vi "Form_设备通讯配置.vi"(11 "Module Admin":refnum<class "lib_QMH_Module_Admin.lvclass">) -> ()   [LabVIEW 2018]
uses:
  Basic Library/Module Admin_class/lib_QMH_Module_Admin.lvclass
  <vilib>/Utility/miscctls.llb/LVPointTypeDef.ctl
  <vilib>/Delacor/Delacor QMH/Libraries/Message Queue_class/Delacor_lib_QMH_Message Queue.lvclass/Delacor_lib_QMH_Message Queue.ctl
  Basic Library/Module Admin_class/lib_QMH_Module_Admin.lvclass/lib_QMH_Module_Admin.ctl
  <vilib>/Delacor/Delacor QMH/Libraries/Message Queue_class/Delacor_lib_QMH_Enqueue Message (Single).vi
  <vilib>/Utility/error.llb/Error Cluster From Error Code.vi
  <vilib>/ErrorRing/Error Ring.xnode
  <vilib>/Delacor/Delacor QMH/Libraries/Message Queue_class/Delacor_lib_QMH_Message Queue.lvclass
  Libraries/DAQ/DAQ.lvlib
panel:
  in  "IP协议":enum32{"IPV4", "IPV6"}(radio)
  in  "Connection Timeout":dbl
  in  "OK":bool caption="确认"
  in  "通信表索引":u16(ring) caption="通信设备" items=["LB-A1", "LB-A2"]
  in  "本机 IP（参考）":string
  in  "设置本机IP":bool
  in  "本机IP下拉列表":u16(ring) caption="本机 IP" items=["192.168.80.1", "192.168.44.1", "192.168.5.160"]
  in  "在网检测":bool caption="通讯检测"
  in  "断线重连":bool=TRUE caption="断线自动重连"
  in  "Protocol":enum16{"Serial Port", "Modbus TCP/IP"}(ring) caption="通讯方式"
  in  "选项卡控件":enum32{"Serial Port", "TCP/IP"}(tab) caption="Serial Settings"
  in  "RS485":T1={"Serial Port"="", "Unit ID"=1, "Baud Rate"=enum."19200", "Mode"=enum."RTU", "Parity"=0} {"Parity" items=["None", "Odd", "Even"]}
  in  "TCP":cluster{"IP Address":string, "Port (502)":u16}={"IP Address"="", "Port (502)"=502}
  in  "Apply":bool caption="应用"
  in  "Cancel":bool caption="取消"
  # "[ms]"
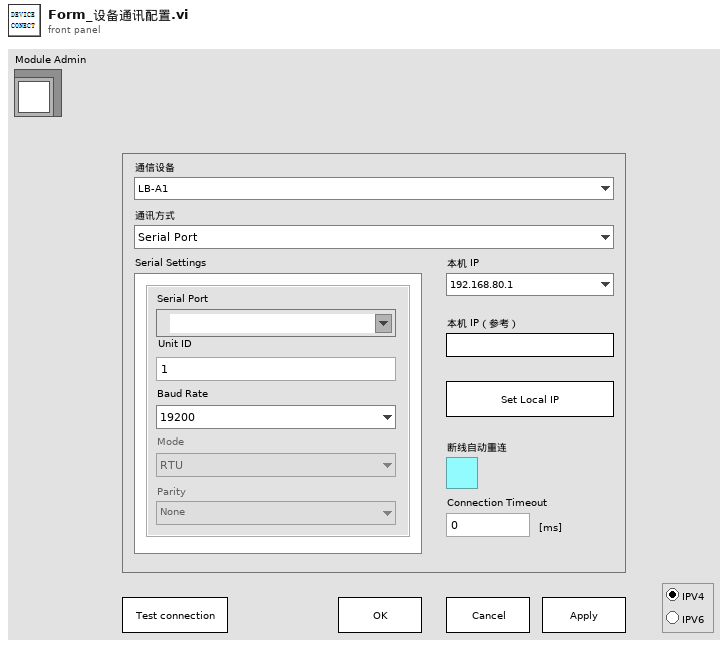
[diagram p1: front panel]
types:
  T1 = cluster{"Serial Port":refnum<visa-resource-name>, "Unit ID":u8, "Baud Rate":enum32{"1200", "2400", "4800", "9600", "19200", "38400", "57600", "115200"}, "Mode":enum16{"RTU", "ASCII"}, "Parity":u16}
  T2 = cluster{"name":string, "appended path":path, "通信表索引":refnum<vi>, "本机IP下拉列表":refnum<vi>, "Protocol":refnum<vi>, "选项卡控件":refnum<vi>, "RS485":refnum<vi>, "TCP":refnum<vi>, "本机 IP（参考）":refnum<vi>, "设置本机IP":refnum<vi>, "断线重连":refnum<vi>}
  T3 = typedef "LVPointTypeDef.ctl" = cluster{"Horizontal":i16, "Vertical":i16}
  T4 = cluster{"COM端口":refnum<visa-resource-name>, "站号":u8, "Baud Rate":enum32{"1200", "2400", "4800", "9600", "19200", "38400", "57600", "115200"}, "串口类型":enum16{"RTU", "ASCII"}, "校验":u16}
  T5 = cluster{"Serial Port":refnum<visa-resource-name>, "Baud Rate":enum32{"1200", "2400", "4800", "9600", "19200", "38400", "57600", "115200"}, "Mode":enum16{"RTU", "ASCII"}, "Parity":u16, "Unit ID":u8, "address":string, "port (502)":u16}
  T6 = enum8{"Enabled", "Disabled", "Disabled and Grayed Out"}
  T7 = cluster{"Unit ID":u8, "IP Address":string, "Port":u16, "Serial Port":string, "baud rate (9600)":u32, "Protocol":enum16{"Serial Port", "Modbus TCP/IP"}}
  T8 = cluster{"设备站号":u8, "IP Addr":string, "Port":u16, "COM":string, "baud rate (9600)":u32, "Protocol":enum16{"Serial Port", "Modbus TCP/IP"}}
  T9 = enum32{"1200", "2400", "4800", "9600", "19200", "38400", "57600", "115200"}
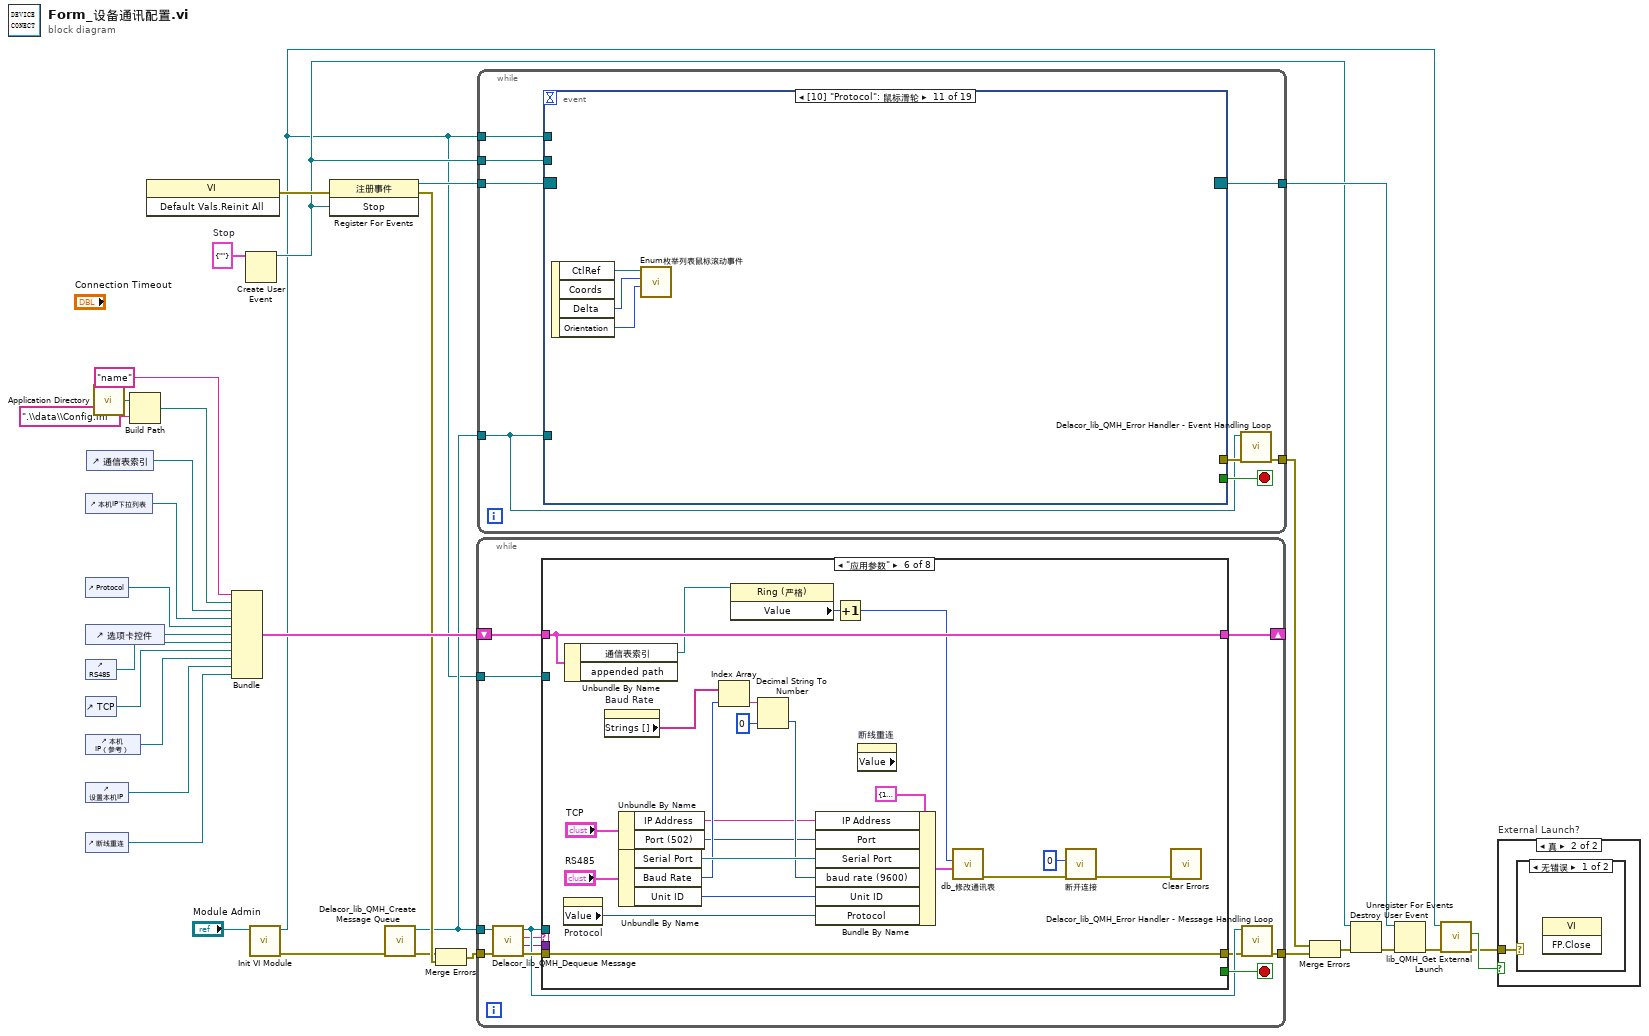
[diagram p0: block diagram]
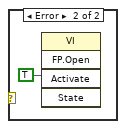
[diagram p3: hidden frame]
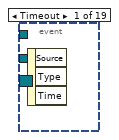
[diagram p4: hidden frame]
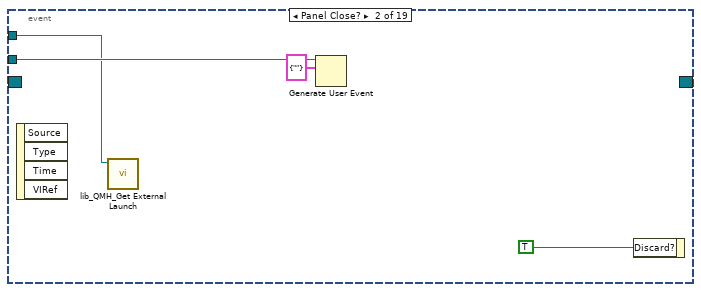
[diagram p5: hidden frame]
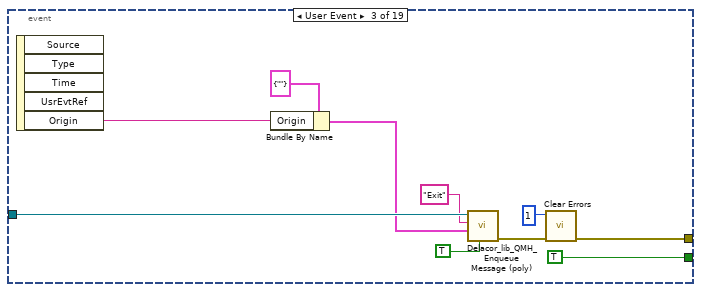
[diagram p6: hidden frame]
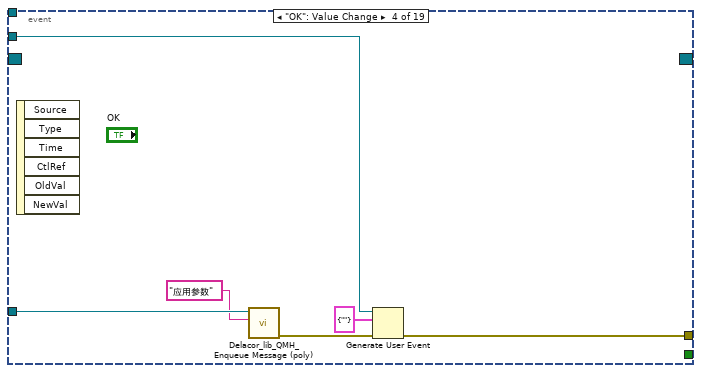
[diagram p7: hidden frame]
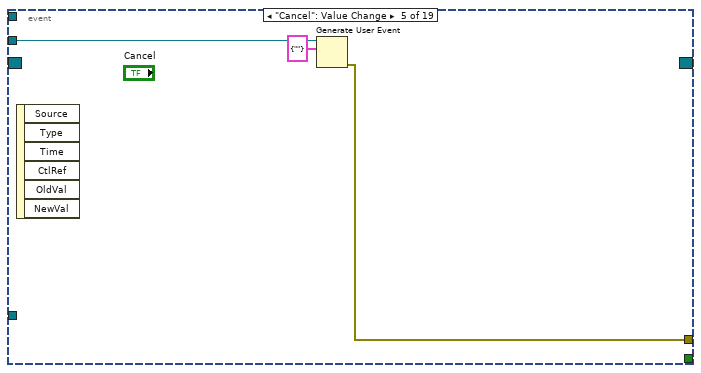
[diagram p8: hidden frame]
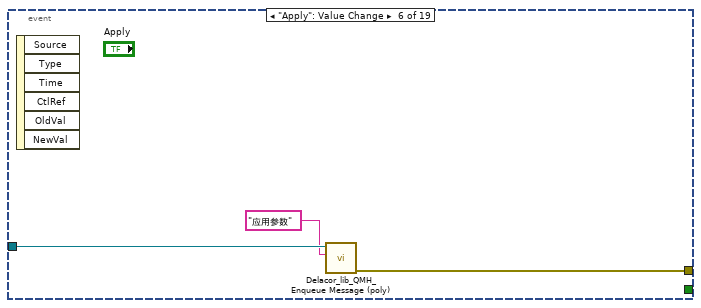
[diagram p9: hidden frame]
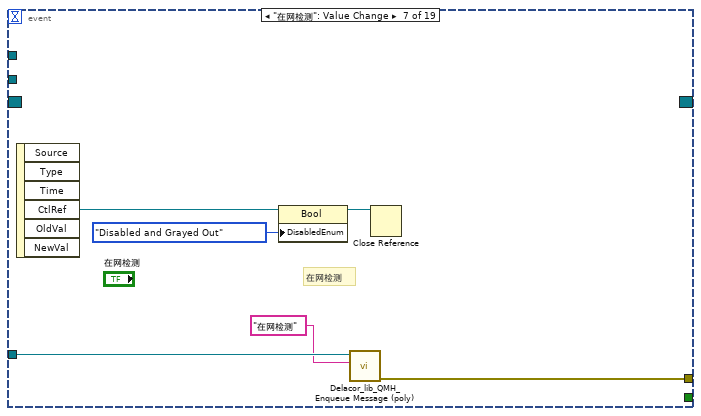
[diagram p10: hidden frame]
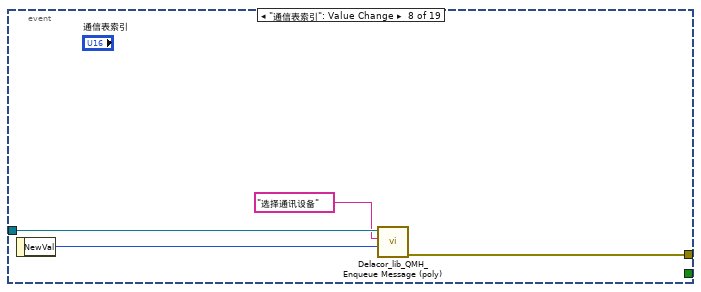
[diagram p11: hidden frame]
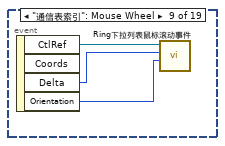
[diagram p12: hidden frame]
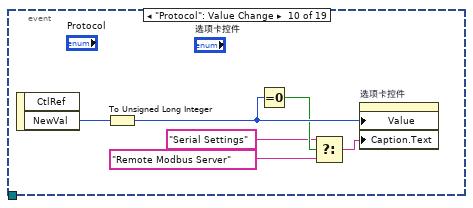
[diagram p13: hidden frame]
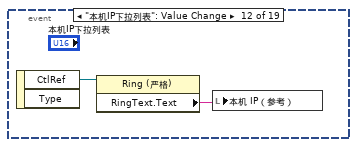
[diagram p14: hidden frame]
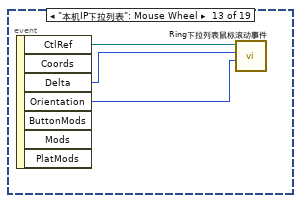
[diagram p15: hidden frame]
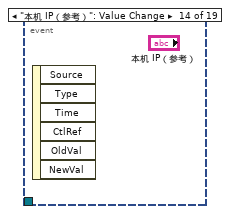
[diagram p16: hidden frame]
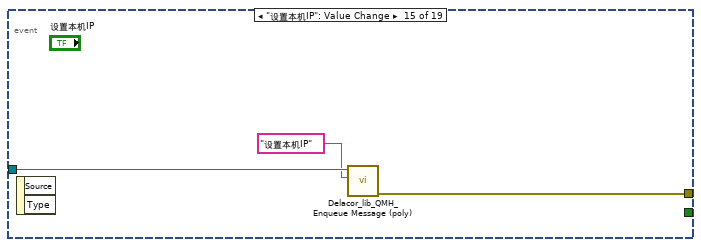
[diagram p17: hidden frame]
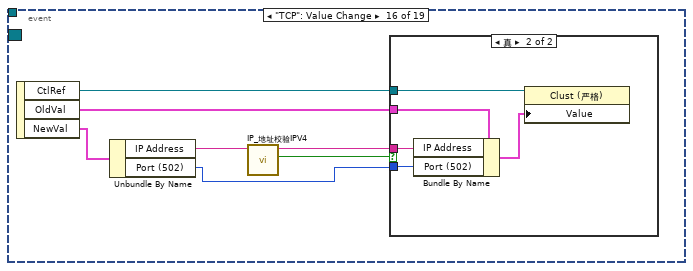
[diagram p18: hidden frame]
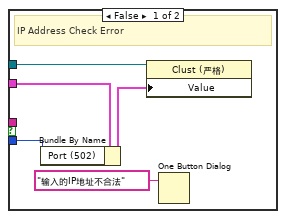
[diagram p19: hidden frame]
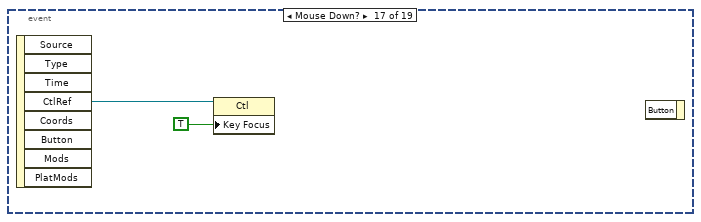
[diagram p20: hidden frame]
diagram:
  w22 = cluster{"Origin":string} {"Origin"=""}  # Stop
  n1 = control-ref of="本机IP下拉列表"() -> (w16:refnum<vi>)
  n2 = control-ref of="Protocol"() -> (w29:refnum<vi>)
  n3 = control-ref of="选项卡控件"() -> (w28:refnum<vi>)
  n4 = control-ref of="RS485"() -> (w27:refnum<vi>)
  n5 = control-ref of="TCP"() -> (w26:refnum<vi>)
  n6 = control-ref of="本机 IP（参考）"() -> (w25:refnum<vi>)
  n7 = control-ref of="设置本机IP"() -> (w24:refnum<vi>)
  n8 = control-ref of="断线重连"() -> (w23:refnum<vi>)
  n9 = control-ref of="通信表索引"() -> (w15:refnum<vi>)
  n10 = call <vilib>:"Application Directory.vi"() -> ("Application Directory"=w13:path)
  n11 = Build Path(base path=w13, name or relative path=".\\data\\Config.ini" ("名称或相对路径")) -> (appended path=w12:path)
  n12 = invoke class="VI" method="Default Vals.Reinit All"() -> (error out=w17:errorcluster)  [unwired: 3 in, 2 out]
  n13 = Bundle("name"="name", "appended path"=w12, "通信表索引"=w15, "本机IP下拉列表"=w16, "Protocol"=w29, "选项卡控件"=w28, "RS485"=w27, "TCP"=w26, "本机 IP（参考）"=w25, "设置本机IP"=w24, "断线重连"=w23) -> (w30:T2)  [unwired: 1 in]
  n14 = Create User Event(user event datatype=w22) -> (user event=w3:refnum<user-event>)  [unwired: 1 in, 1 out]
  n15 = call "Init VI Module.vi"("Module Admin in"="Module Admin") -> ("error out"=w11:errorcluster, "Module Admin out"=w2:refnum<class "lib_QMH_Module_Admin.lvclass">)  [unwired: 9 in]
  n16 = register-events(error in=w17, w3) -> (reference out=w31:refnum<event-registration>, error out=w20:errorcluster)  [unwired: 1 in]
  n17 = call <vilib>:"Delacor_lib_QMH_Create Message Queue.vi"("error in"=w11) -> ("error out"=w18:errorcluster, "Message Queue"=w19:refnum<class "Delacor_lib_QMH_Message Queue.lvclass">)  [unwired: 9 in]
  n18 = Merge Errors(w18, w20) -> (w21:errorcluster)
  n19 = while {
    tunnel: w19 -> [w41]
    tunnel: w21 -> [w42]
    tunnel: [w35] -> w33
    shift-right: [w44] -> _
    shift-left: w30 -> [w43]
    tunnel: w2 -> [w34]
    stop <- w45 stop-if-true
    n20 = call-dynamic "Delacor_lib_QMH_Dequeue Message.vi"("error in"=w42, "Message Queue in"=w41) -> ("error out"=w40:errorcluster, "Message Data"=w37:variant, "Message"=w38:string, "Message Queue out"=w39:refnum<class "Delacor_lib_QMH_Message Queue.lvclass">)  [unwired: 6 in]
    n21 = case shown="\"应用参数\"" w38 {
      selector: w38 -> [w50 _ _ _ _ _ _ _]
      tunnel: w39 -> [_ w64 _ _ _ _ w162 w172]
      tunnel: w40 -> [w47 w63 w101 w106 w136 w156 w167 w177]
      tunnel: w37 -> [_ _ w99 _ _ _ w168 w178]
      tunnel: [_ _ _ _ _ _ _ TRUE] -> w45
      tunnel: [w46 w62 w100 w106 w136 w156 w163 w171] -> w36
      tunnel: [w49 w73 w97 w102 w135 w158 w169 w173] -> w44
      tunnel: w43 -> [w49 w73 w97 w102 w135 w158 w169 w173]
      tunnel: w34 -> [_ _ _ _ _ _ _ _]
      frame "", Default {
        n22 = Unbundle By Name(w49) -> ("name"=w48:string)
        n23 = xnode "错误下拉列表"("参数 0"=w50, "参数 1"=w48) -> ("错误输出"=w51:errorcluster)
        n24 = Merge Errors(w47, w51) -> (w46:errorcluster)
      }
      frame "Initialize" {
        w60 = u16 0 ("值")
        n25 = Unbundle By Name(w73) -> ("本机IP下拉列表"=w72:refnum<vi>, "本机 IP（参考）"=w68:refnum<vi>, "通信表索引"=w66:refnum<vi>)
        n26 = String To IP(1:"" ("名称")) -> (0:w70:u32[])
        n27 = call "db_查询通讯设备名称列表.vi"() -> ("通讯设备列表名"=w65:string[])  [unwired: 10 in, 1 out]
        n28 = for {
          tunnel: w70 -> [w77] mode=indexing
          tunnel: [w75] -> w69 mode=indexing
          n29 = IP To String(1:TRUE ("句点符号？(F)"), 2:w77) -> (0:w75:string)
        }
        n30 = property class="Ring (严格)"(reference=w66, "Strings []"=w65, "Value"=w60) -> ()  [unwired: 1 in, 2 out]
        n31 = call-poly <vilib>:"Delacor_lib_QMH_Enqueue Message (poly).vi"("error in"=w63, "Message Data"=w60, "Message"="选择通讯设备", "Message Queue in"=w64) -> ("error out"=w62:errorcluster)  [unwired: 6 in, 1 out]
        n32 = property class="Ring (严格)"(reference=w72, "Strings []"=w69) -> ("RingText.Text"=w67:string)  [unwired: 1 in, 2 out]
        n33 = property class="Str"(reference=w68, "Text.Text"=w67) -> ()  [unwired: 1 in, 2 out]
        n34 = property on="窗格" class="Pane"("Origin"=T3 {"Horizontal"=0, "Vertical"=0} ("原点")) -> ()  [unwired: 2 in, 2 out]
      }
      frame "选择通讯设备" {
        n35 = Unbundle By Name(w97) -> ("TCP"=w96:refnum<vi>, "RS485"=w95:refnum<vi>, "Protocol"=w94:refnum<vi>)  [unwired: 1 out]
        n36 = Variant To Data(error in=w101, type=0, Variant=w99) -> (data=w88:i32, error out=w100:errorcluster)
        n37 = Increment(x=w88) -> (x+1=w82:i32)
        n38 = property on="Baud Rate" class="Enum (严格)"() -> ("Strings []"=w92:string[])  [unwired: 2 in, 2 out]
        n39 = call "db_查询通讯表.vi"("ID"=w82) -> ("设备通讯参数"=w87:T8)  [unwired: 9 in, 1 out]
        n40 = Unbundle By Name(w87) -> ("IP Addr"=w78:string, "Port"=w80:u16, "COM"=w93:string, "baud rate (9600)"=w91:u32, "设备站号"=w85:u8, "Protocol"=w86:enum16{"Serial Port", "Modbus TCP/IP"})
        n41 = Number To Decimal String(number=w91) -> (decimal integer string=w90:string)  [unwired: 1 in]
        n42 = Search 1D Array(1D array=w92, element=w90) -> (index of element=w89:i32)  [unwired: 1 in]
        n43 = Bundle By Name(cluster=cluster{"IP Address":string, "Port (502)":u16} {"IP Address"="", "Port (502)"=0} ("值"), "IP Address"=w78, "Port (502)"=w80) -> (w81:cluster{"IP Address":string, "Port (502)":u16})
        n44 = Bundle By Name(cluster=T4 {"COM端口"="", "站号"=0, "Baud Rate"=enum."1200", "串口类型"=enum."RTU", "校验"=0} ("值"), "COM端口"=w93, "Baud Rate"=w89, "站号"=w85) -> (w83:T4)
        n45 = property on="属性节点" class="Enum (严格)"(reference=w94, "Val(Sgnl)"=w86) -> ()  [unwired: 1 in, 2 out]
        n46 = property class="Clust (严格)"(reference=w95, "Value"=w83) -> ()  [unwired: 1 in, 2 out]
        n47 = property class="Clust (严格)"(reference=w96, "Value"=w81) -> ()  [unwired: 1 in, 2 out]
      }
      frame "设置本机IP" {
        n48 = Unbundle By Name(w102) -> ("本机 IP（参考）"=w105:refnum<vi>)
        n49 = property class="Str"(reference=w105) -> ("Value"=w104:string)  [unwired: 1 in, 2 out]
        n50 = call "IP_设置本机IP地址.vi"("IP模式"=enum16{"使用特定ip", "自动获取ip"}."使用特定ip", "IP Address"=w104) -> ()  [unwired: 7 in, 3 out]
      }
      frame "在网检测" {
        w127 = 128  # call and forget
        n51 = Unbundle By Name(w135) -> ("Protocol"=w134:refnum<vi>, "RS485"=w133:refnum<vi>, "TCP"=w132:refnum<vi>)
        n52 = property on="属性节点" class="Clust (严格)"(reference=w133) -> ("Value"=w116:T1)  [unwired: 1 in, 2 out]
        n53 = property on="属性节点" class="Clust (严格)"(reference=w132) -> ("Value"=w130:cluster{"IP Address":string, "Port (502)":u16})  [unwired: 1 in, 2 out]
        n54 = property on="属性节点" class="Enum (严格)"(reference=w134) -> ("Value"=w120:enum16{"Serial Port", "Modbus TCP/IP"})  [unwired: 1 in, 2 out]
        n55 = Unbundle By Name(w130) -> ("IP Address"=w110:string, "Port (502)"=w117:u16)
        n56 = Unbundle By Name(w116) -> ("Serial Port"=w113:refnum<visa-resource-name>, "Unit ID"=w112:u8, "Baud Rate"=w114:T9, "Mode"=w111:enum16{"RTU", "ASCII"}, "Parity"=w115:u16)
        n57 = vi-ref "Modbus Connection Test.vi"() -> (w121:refnum<vi>)
        n58 = Bundle By Name(cluster=T5 {"Serial Port"="", "Baud Rate"=enum."1200", "Mode"=enum."RTU", "Parity"=0, "Unit ID"=0, "address"="", "port (502)"=0} ("Modbus Info"), "Serial Port"=w113, "Baud Rate"=w114, "Mode"=w111, "Parity"=w115, "Unit ID"=w112, "address"=w110, "port (502)"=w117) -> (w118:T5)
        n59 = property class="VI"(reference=w121) -> (reference out=w109:refnum<vi>, error out=w128:errorcluster, "Path"=w129:path)  [unwired: 1 in]
        n60 = Open VI Reference(type specifier VI Refnum (for type only)=refnum<vi> refnum, vi path=w129, options=w127, error in (no error)=w128) -> (vi reference=w124:refnum<vi>, error out=w125:errorcluster)  [unwired: 2 in]
        n61 = call-by-ref "Start Asynchronous Call"(reference=w124, error in=w125, "Protocol"=w120, "Modbus Info"=w118) -> (reference out=w123:refnum<vi>, error out=w122:errorcluster)  [unwired: 9 in, 1 out]
        n62 = Close Reference(reference=w123, error in (no error)=w122) -> (error out=w108:errorcluster)
        n63 = Close Reference(reference=w109, error in (no error)=w108) -> (error out=w107:errorcluster)
        n64 = property on="在网检测" class="Bool"(error in=w107, "DisabledEnum"=T6."Enabled" ("禁用")) -> ()  [unwired: 1 in, 2 out]
      }
      frame "应用参数" {
        n65 = property on="Protocol" class="Enum (严格)"() -> ("Value"=w152:enum16{"Serial Port", "Modbus TCP/IP"})  [unwired: 2 in, 2 out]
        n66 = Unbundle By Name(w158) -> ("通信表索引"=w155:refnum<vi>)  [unwired: 1 out]
        n67 = property on="Baud Rate" class="Enum (严格)"() -> ("Strings []"=w148:string[])  [unwired: 2 in, 2 out]
        n68 = Unbundle By Name("TCP") -> ("IP Address"=w140:string, "Port (502)"=w143:u16)
        n69 = Unbundle By Name("RS485") -> ("Serial Port"=w154:refnum<visa-resource-name>, "Baud Rate"=w147:T9, "Unit ID"=w151:u8)
        n70 = Index Array(array=w148, index=w147) -> (element=w146:string)
        n71 = property class="Ring (严格)"(reference=w155) -> ("Value"=w144:u16)  [unwired: 1 in, 2 out]
        n72 = Decimal String To Number(string=w146, default (0L)=u32 0 ("默认(0 I32)")) -> (number=w149:u32)  [unwired: 1 in, 1 out]
        n73 = Bundle By Name(cluster=T7 {"Unit ID"=1, "IP Address"="127.0.0.1", "Port"=255, "Serial Port"="COM3", "baud rate (9600)"=9600, "Protocol"=enum."Serial Port"} ("设备通讯参数"), "IP Address"=w140, "Port"=w143, "Serial Port"=w154, "baud rate (9600)"=w149, "Unit ID"=w151, "Protocol"=w152) -> (w141:T7)
        n74 = Increment(x=w144) -> (x+1=w145:u16)
        n75 = property on="断线重连" class="Bool (严格)" props=["Value"]() -> ()  [unwired: 2 in, 3 out]
        n76 = call "db_修改通讯表.vi"("设备通讯参数"=w141, "id"=w145) -> ("error out"=w138:errorcluster)  [unwired: 8 in, 1 out]
        n77 = call "断开连接.vi"("error in"=w138, "Mod ID"=0) -> ("error out"=w137:errorcluster)  [unwired: 9 in]
        n78 = call <vilib>:"Clear Errors.vi"("error in (no error)"=w137) -> ()  [unwired: 5 in, 2 out]
      }
      frame "Error" {
        n79 = Variant To Data(error in=w167, type=errorcluster {"status"=FALSE, "code"=0, "source"=""} ("error constant"), Variant=w168) -> (data=w165:errorcluster, error out=w164:errorcluster)
        n80 = call <vilib>:"Simple Error Handler.vi"("error in (no error)"=w165) -> ()  [unwired: 4 in, 5 out]
        n81 = call-poly <vilib>:"Delacor_lib_QMH_Enqueue Message (poly).vi"("Priority Message? (F)"=TRUE, "Message"="Exit", "Message Queue in"=w162) -> ("error out"=w161:errorcluster)  [unwired: 7 in, 1 out]
        n82 = Merge Errors(w164, w161) -> (w163:errorcluster)
      }
      frame "Exit" {
        w179 = 91  # 91: not all Exit messages will have an argument
        n83 = Variant To Data(error in=w177, type=cluster{"Origin":string} {"Origin"=""}, Variant=w178) -> (data=w174:cluster{"Origin":string}, error out=w176:errorcluster)
        n84 = Unbundle By Name(w174) -> ()  [unwired: 1 out]
        n85 = call <vilib>:"Clear Errors.vi"("error in (no error)"=w176, "specific error code to clear (0: all)"=w179) -> ("error out"=w170:errorcluster)  [unwired: 4 in, 1 out]
        n86 = call-dynamic "Delacor_lib_QMH_Release Message Queue.vi"("error in"=w170, "Message Queue"=w172) -> ("error out"=w171:errorcluster)  [unwired: 9 in]
      }
    }
    n87 = call-dynamic "Delacor_lib_QMH_Error Handler - Message Handling Loop.vi"("error in"=w36, "Message Queue in"=w39) -> ("dup error in"=w35:errorcluster)  [unwired: 8 in, 1 out]
  }
  n88 = while {
    tunnel: w19 -> [w183]
    tunnel: [w182] -> w32
    tunnel: [w187] -> w4
    tunnel: w31 -> [w186]
    tunnel: w3 -> [w185]
    tunnel: w2 -> [w181]
    stop <- w188 stop-if-true
    n89 = event shown="[10] \"Protocol\": 鼠标滑轮" {
      selector: w186 -> [_ _ _ _ _ _ _ _ _ _ _ _ _ _ _ _ _ _ _]
      dyn-events: [_ _ _ _ _ _ _ _ _ _ _ _ _ _ _ _ _ _ _] -> w187
      timeout: _ -> [_ _ _ _ _ _ _ _ _ _ _ _ _ _ _ _ _ _ _]
      tunnel: [_ _ TRUE ("放弃？") _ _ _ _ _ _ _ _ _ _ _ _ _ _ _ _] -> w188
      tunnel: w183 -> [_ _ w197 w204 _ w214 w220 w224 _ _ _ _ _ _ w244 _ _ _ _]
      tunnel: [_ _ w200 w205 w209 w213 w219 w223 _ _ _ _ _ _ w243 _ _ _ _] -> w184
      tunnel: w185 -> [_ w191 _ w207 w211 _ _ _ _ _ _ _ _ _ _ _ _ _ _]
      tunnel: w181 -> [_ w189 _ _ _ _ _ _ _ _ _ _ _ _ _ _ _ _ _]
      event Timeout {
        n90 = event-data() -> ()  [unwired: 1 in, 3 out]
      }
      event Panel Close? {
        n91 = event-data() -> ()  [unwired: 1 in, 4 out]
        n92 = call "lib_QMH_Get External Launch.vi"("Module Admin in"=w189) -> ()  [unwired: 8 in, 3 out]
        n93 = Generate User Event(user event=w191, event data cluster=cluster{"Origin":string} {"Origin"=""} ("事件数据")) -> ()  [unwired: 2 in, 2 out]
        n94 = event-data("Discard?"=TRUE ("放弃？")) -> ()  [unwired: 1 in, 1 out]
      }
      event User Event {
        n95 = event-data() -> ("Origin"=w198:string)  [unwired: 1 in, 4 out]
        n96 = Bundle By Name(cluster=cluster{"Origin":string} {"Origin"=""}, "Origin"=w198) -> (w195:cluster{"Origin":string})
        n97 = call-poly <vilib>:"Delacor_lib_QMH_Enqueue Message (poly).vi"("Priority Message? (F)"=TRUE, "Message Data"=w195, "Message"="Exit", "Message Queue in"=w197) -> ("error out"=w193:errorcluster)  [unwired: 6 in, 1 out]
        n98 = call <vilib>:"Clear Errors.vi"("error in (no error)"=w193, "specific error code to clear (0: all)"=1) -> ("error out"=w200:errorcluster)  [unwired: 4 in, 1 out]
      }
      event "OK": Value Change {
        n99 = event-data() -> ()  [unwired: 1 in, 6 out]
        n100 = call-poly <vilib>:"Delacor_lib_QMH_Enqueue Message (poly).vi"("Message"="应用参数", "Message Queue in"=w204) -> ("error out"=w206:errorcluster)  [unwired: 8 in, 1 out]
        n101 = Generate User Event(user event=w207, event data cluster=cluster{"Origin":string} {"Origin"=""} ("事件数据"), error in=w206) -> (error out=w205:errorcluster)  [unwired: 1 in, 1 out]
      }
      event "Cancel": Value Change {
        n102 = event-data() -> ()  [unwired: 1 in, 6 out]
        n103 = Generate User Event(user event=w211, event data cluster=cluster{"Origin":string} {"Origin"=""} ("事件数据")) -> (error out=w209:errorcluster)  [unwired: 2 in, 1 out]
      }
      event "Apply": Value Change {
        n104 = event-data() -> ()  [unwired: 1 in, 6 out]
        n105 = call-poly <vilib>:"Delacor_lib_QMH_Enqueue Message (poly).vi"("Message"="应用参数", "Message Queue in"=w214) -> ("error out"=w213:errorcluster)  [unwired: 8 in, 1 out]
      }
      event "在网检测": Value Change {
        # "在网检测"
        n106 = event-data() -> ("CtlRef"=w216:refnum<vi>)  [unwired: 1 in, 5 out]
        n107 = property on="属性节点" class="Bool"(reference=w216, "DisabledEnum"=T6."Disabled and Grayed Out" ("禁用")) -> (reference out=w215:refnum<vi>)  [unwired: 1 in, 1 out]
        n108 = call-poly <vilib>:"Delacor_lib_QMH_Enqueue Message (poly).vi"("Message"="在网检测", "Message Queue in"=w220) -> ("error out"=w219:errorcluster)  [unwired: 8 in, 1 out]
        n109 = Close Reference(reference=w215) -> ()  [unwired: 1 in, 1 out]
      }
      event "通信表索引": Value Change {
        n110 = event-data() -> ("NewVal"=w221:u16)  [unwired: 1 in]
        n111 = call-poly <vilib>:"Delacor_lib_QMH_Enqueue Message (poly).vi"("Message Data"=w221, "Message"="选择通讯设备", "Message Queue in"=w224) -> ("error out"=w223:errorcluster)  [unwired: 7 in, 1 out]
      }
      event "通信表索引": Mouse Wheel {
        n112 = event-data() -> ("CtlRef"=w227:refnum<vi>, "Delta"=w226:i32, "Orientation"=w225:enum16{"Horizontal", "Vertical"})  [unwired: 1 in, 1 out]
        n113 = call "Ring下拉列表鼠标滚动事件.vi"("方向"=w225, "Delta"=w226, "CtlRef"=w227) -> ()  [unwired: 7 in, 2 out]
      }
      event "Protocol": Value Change {
        n114 = event-data() -> ("NewVal"=w233:enum16{"Serial Port", "Modbus TCP/IP"})  [unwired: 1 in, 1 out]
        n115 = To Unsigned Long Integer(number=w233) -> (unsigned 32bit integer=w232:u32)
        n116 = Equal To 0?(x=w232) -> (x = 0?=w231:bool)
        n117 = Select(t="Serial Settings" ("标题.文本"), s=w231, f="Remote Modbus Server" ("标题.文本")) -> (s? t:f=w228:string)
        n118 = property on="选项卡控件" class="TabCtl (严格)"("Value"=w232, "Caption.Text"=w228) -> ()  [unwired: 2 in, 2 out]
      }
      event "Protocol": Mouse Wheel {
        n119 = event-data() -> ("CtlRef"=w236:refnum<vi>, "Delta"=w235:i32, "Orientation"=w234:enum16{"Horizontal", "Vertical"})  [unwired: 1 in, 1 out]
        n120 = call "Enum枚举列表鼠标滚动事件.vi"("方向"=w234, "Delta"=w235, "CtlRef"=w236) -> ()  [unwired: 7 in, 2 out]
      }
      event "本机IP下拉列表": Value Change {
        n121 = event-data() -> ("CtlRef"=w238:refnum<vi>)  [unwired: 1 in, 1 out]
        n122 = property class="Ring (严格)"(reference=w238) -> ("RingText.Text"=w237:string)  [unwired: 1 in, 2 out]
        n123 = local write "本机 IP（参考）"(w237) -> ()
      }
      event "本机IP下拉列表": Mouse Wheel {
        n124 = event-data() -> ("CtlRef"=w241:refnum<vi>, "Delta"=w240:i32, "Orientation"=w239:enum16{"Horizontal", "Vertical"})  [unwired: 1 in, 4 out]
        n125 = call "Ring下拉列表鼠标滚动事件.vi"("方向"=w239, "Delta"=w240, "CtlRef"=w241) -> ()  [unwired: 7 in, 2 out]
      }
      event "本机 IP（参考）": Value Change {
        n126 = event-data() -> ()  [unwired: 1 in, 6 out]
      }
      event "设置本机IP": Value Change {
        n127 = event-data() -> ()  [unwired: 1 in, 2 out]
        n128 = call-poly <vilib>:"Delacor_lib_QMH_Enqueue Message (poly).vi"("Message"="设置本机IP", "Message Queue in"=w244) -> ("error out"=w243:errorcluster)  [unwired: 8 in, 1 out]
      }
      event "TCP": Value Change {
        n129 = event-data() -> ("CtlRef"=w246:refnum<vi>, "OldVal"=w249:cluster{"IP Address":string, "Port (502)":u16}, "NewVal"=w251:cluster{"IP Address":string, "Port (502)":u16})  [unwired: 1 in]
        n130 = Unbundle By Name(w251) -> ("IP Address"=w250:string, "Port (502)"=w245:u16)
        n131 = call "IP_地址校验IPV4.vi"("IP Address"=w250) -> ("合法？"=w248:bool, "所有匹配"=w247:string)  [unwired: 9 in]
        n132 = case shown="真" w248 {
          tunnel: w246 -> [w256 w261]
          tunnel: w249 -> [w255 w260]
          tunnel: w247 -> [_ w258]
          tunnel: w245 -> [w252 w257]
          frame False {
            # "IP Address Check Error"
            n133 = Bundle By Name(cluster=w255, "Port (502)"=w252) -> (w253:cluster{"IP Address":string, "Port (502)":u16})
            n134 = property class="Clust (严格)"(reference=w256, "Value"=w253) -> ()  [unwired: 1 in, 2 out]
            n135 = One Button Dialog(message="输入的IP地址不合法" ("消息")) -> ()  [unwired: 1 in, 1 out]
          }
          frame True {
            n136 = Bundle By Name(cluster=w260, "IP Address"=w258, "Port (502)"=w257) -> (w259:cluster{"IP Address":string, "Port (502)":u16})
            n137 = property class="Clust (严格)"(reference=w261, "Value"=w259) -> ()  [unwired: 1 in, 2 out]
          }
        }
      }
      event "TCP.IP Address", "TCP.Port (502)": Mouse Down? {
        n138 = event-data() -> ("CtlRef"=w262:refnum<vi>)  [unwired: 1 in, 7 out]
        n139 = property class="Ctl"(reference=w262, "Key Focus"=TRUE ("键选中")) -> ()  [unwired: 1 in, 2 out]
        n140 = event-data() -> ()  [unwired: 2 in, 1 out]
      }
      event "TCP.IP Address", "TCP.Port (502)": Mouse Move {
        n141 = event-data() -> ()  [unwired: 1 in, 5 out]
      }
      event "断线重连": Value Change {
        n142 = event-data() -> ()  [unwired: 1 in, 2 out]
      }
    }
    n143 = call-dynamic "Delacor_lib_QMH_Error Handler - Event Handling Loop.vi"("error in"=w184, "Message Queue in"=w183) -> ("dup error in"=w182:errorcluster)  [unwired: 8 in, 1 out]
  }
  n144 = Merge Errors(w32, w33) -> (w5:errorcluster)
  n145 = Destroy User Event(user event=w3, error in=w5) -> (error out=w9:errorcluster)
  n146 = Unregister For Events(event registration refnum=w4, error in=w9) -> (error out=w8:errorcluster)
  n147 = call "lib_QMH_Get External Launch.vi"("error in (no error)"=w8, "Module Admin in"=w2) -> ("error out"=w6:errorcluster, "External Launch"=w7:bool)  [unwired: 7 in, 1 out]
  n148 = case "External Launch?" shown="真" w7 {
    tunnel: w6 -> [_ w264]
    frame False {
    }
    frame True {
      n149 = case "条件结构" shown="无错误" w264 {
        frame No Error {
          n150 = invoke class="VI" method="FP.Close"() -> ()  [unwired: 3 in, 3 out]
        }
        frame Error {
          n151 = invoke class="VI" method="FP.Open"("Activate"=TRUE ("Activate?")) -> ()  [unwired: 4 in, 5 out]
        }
      }
    }
  }
